vi "GenerateStimulusOutputs_Optogenetics.vi"(0 "Trial duration (min)":dbl, 1 "Rest duration(s)":dbl, 2 "trial offset (s)":dbl, 3 "Left Pad":dbl, 4 "Right Pad":dbl, 5 "Auditory":dbl, 6 "LED":dbl, 8 "LED Stim Duration (s)":dbl, 9 "LED Stim Parameters":cluster{"Fs":dbl, "Samples":dbl}, 10 "LED Frequency":dbl, 11 "Sol Stim Parameters":cluster{"Fs":dbl, "Samples":dbl}, 12 "LED duty cycle (%)":dbl, 14 "Sol Stim Duration (s)":dbl, 16 "Sol Frequency":dbl, 18 "Sol Duty Cycle (%)":dbl) -> (15 "Double LED Out":dbl[](array[numeric]), 20 "Solenoid Stim Waveforms":digitalwaveform(graph), 22 "Stimulus Digital Outputs":digitalwaveform[](array[waveform]), 24 "Left Pad Out":digitalwaveform(graph), 25 "Auditory Out":digitalwaveform(graph), 26 "Right Pad Out":digitalwaveform(graph), 27 "LED Out":digitalwaveform(graph))   [LabVIEW 2018]
uses:
  <vilib>/Waveform/DWDTOps.llb/DWDT Analog to Digital.vi
  <vilib>/Waveform/DWDTOps.llb/DWDT Digital to Analog.vi
  <vilib>/measure/NI_MABase.lvlib
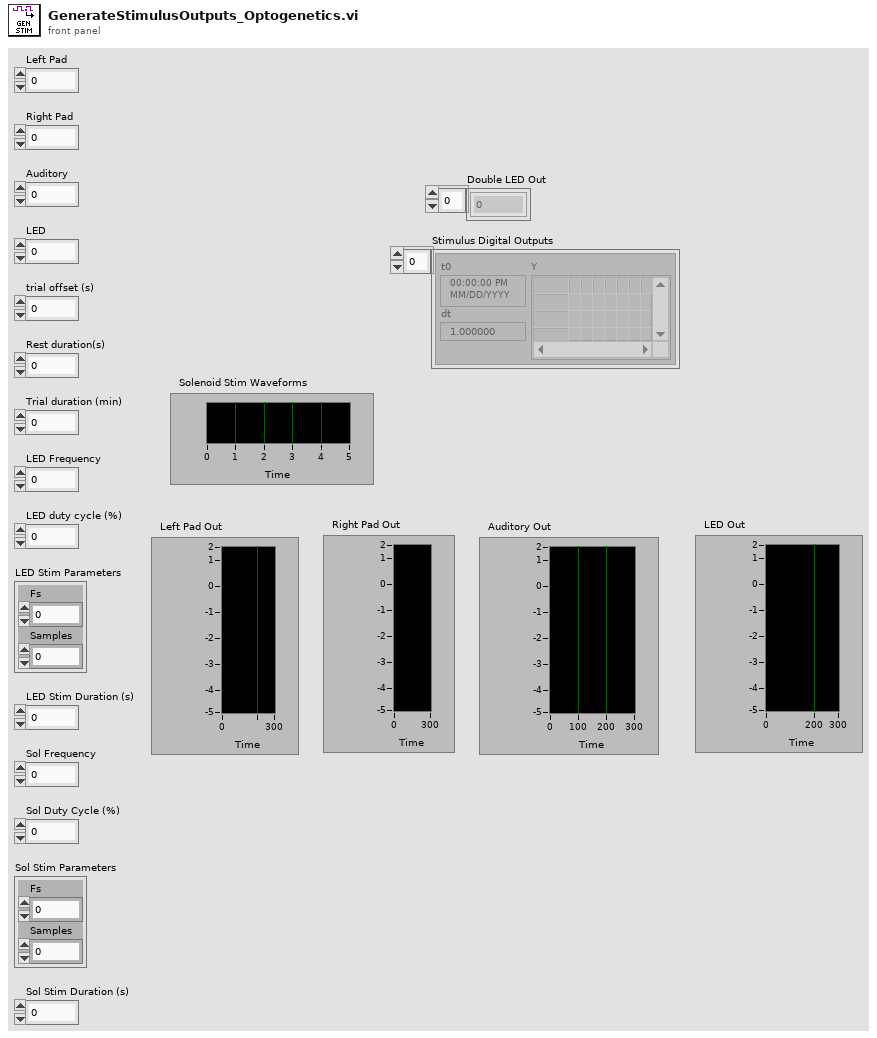
[diagram p1: front panel]
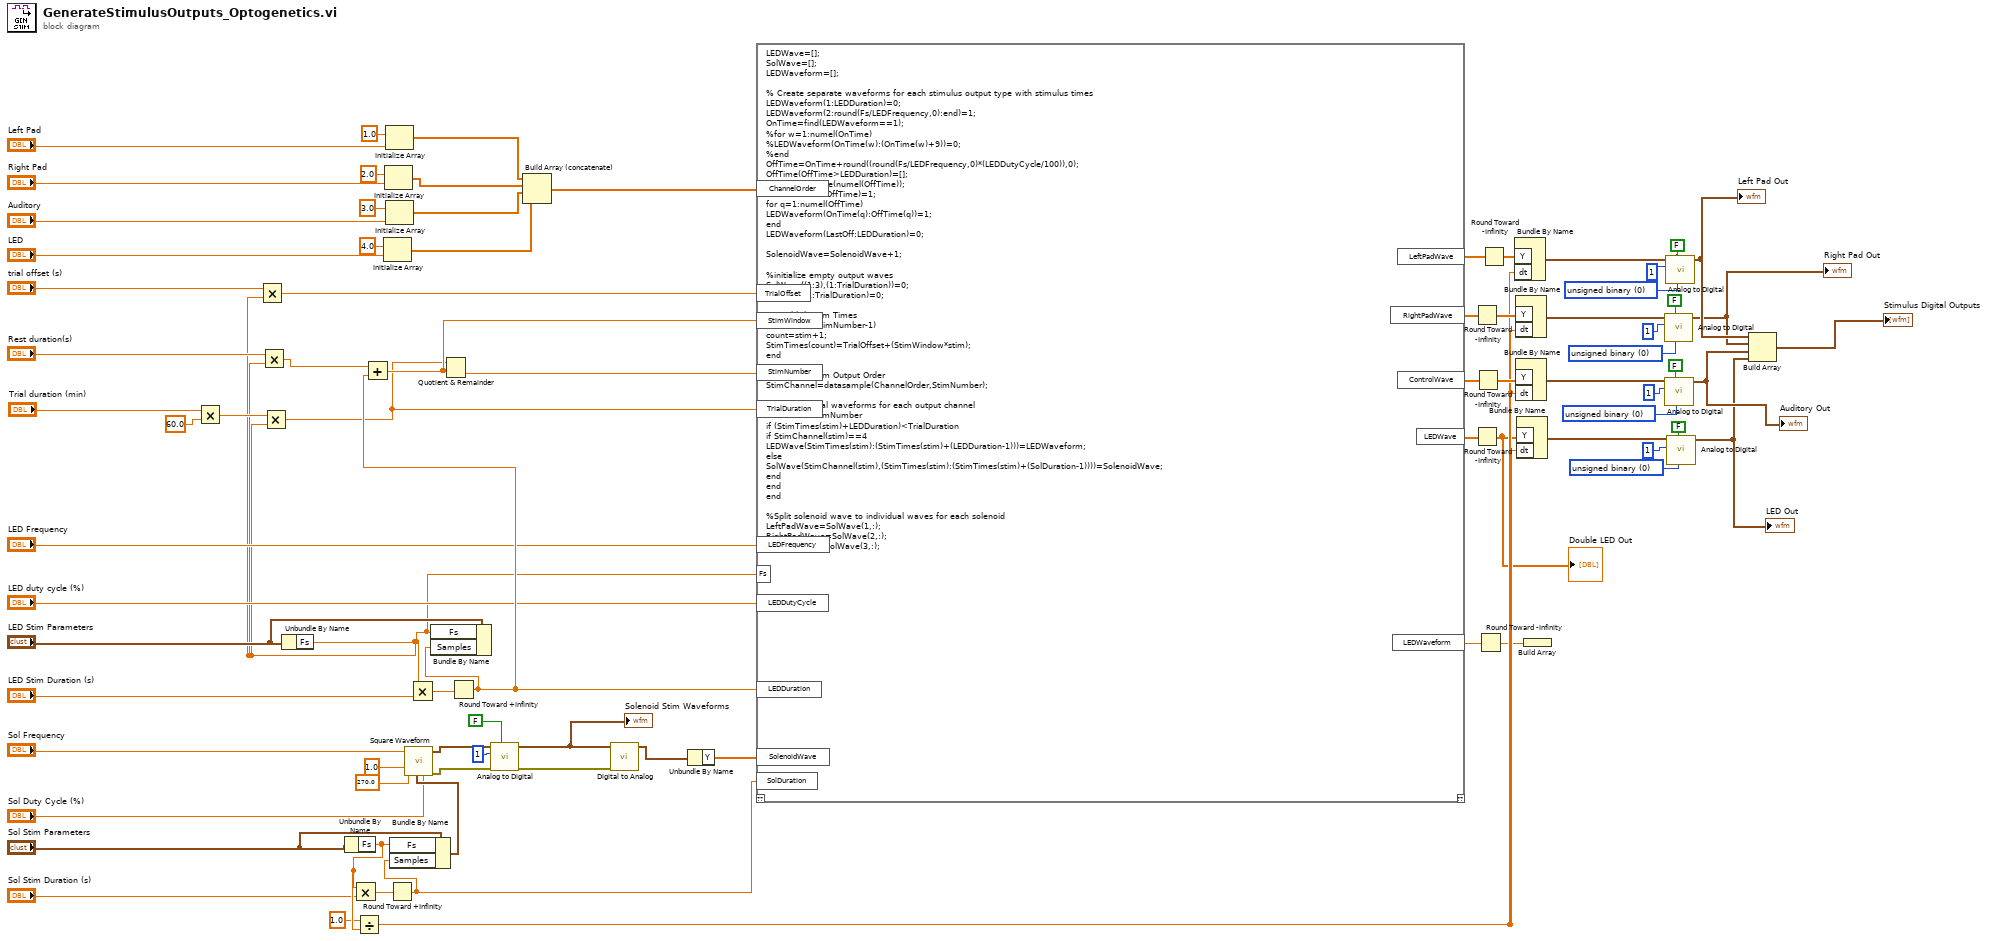
[diagram p0: block diagram]
diagram:
  w78 = u16 0 items=["unsigned binary", "offset binary", "2's complement"] ("data format (offset binary)")
  w77 = u16 0 items=["unsigned binary", "offset binary", "2's complement"] ("data format (offset binary)")
  w76 = u16 0 items=["unsigned binary", "offset binary", "2's complement"] ("data format (offset binary)")
  w75 = u16 0 items=["unsigned binary", "offset binary", "2's complement"] ("data format (offset binary)")
  n1 = Multiply(x="Trial duration (min)", y=60.0) -> (x*y=w16:dbl)
  n2 = Unbundle By Name("LED Stim Parameters") -> ("Fs"=w8:dbl)
  n3 = Multiply(x="trial offset (s)", y=w8) -> (x*y=w63:dbl)
  n4 = Multiply(x="Rest duration(s)", y=w8) -> (x*y=w20:dbl)
  n5 = Multiply(x=w16, y=w8) -> (x*y=w4:dbl)
  n6 = Unbundle By Name("Sol Stim Parameters") -> ("Fs"=w68:dbl)
  n7 = Multiply(x=w68, y="Sol Stim Duration (s)") -> (x*y=w50:dbl)
  n8 = Divide(x=1.0, y=w68) -> (x/y=w7:dbl)
  n9 = Initialize Array(4.0 ("element"), "LED") -> (w32:dbl[])
  n10 = Initialize Array(2.0 ("element"), "Right Pad") -> (w30:dbl[])
  n11 = Initialize Array(1.0 ("element"), "Left Pad") -> (w29:dbl[])
  n12 = Initialize Array(3.0 ("element"), "Auditory") -> (w31:dbl[])
  n13 = Round Toward +Infinity(x=w50) -> (ceil(x): smallest int >= x=w51:dbl)
  n14 = Bundle By Name(cluster="Sol Stim Parameters", "Fs"=w68, "Samples"=w51) -> (w38:cluster{"Fs":dbl, "Samples":dbl})
  n15 = call <vilib>:"Square Waveform.vi"("duty cycle (%)"="Sol Duty Cycle (%)", "sampling info"=w38, "phase"=270.0, "amplitude"=1.0, "frequency"="Sol Frequency") -> ("error out"=w41:errorcluster, "signal out"=w44:waveform(dbl))  [unwired: 5 in]
  n16 = Multiply(x=w8, y="LED Stim Duration (s)") -> (x*y=w49:dbl)
  n17 = Round Toward +Infinity(x=w49) -> (ceil(x): smallest int >= x=w80:dbl)
  n18 = Add(x=w20, y=w80) -> (x+y=w64:dbl)
  n19 = Bundle By Name(cluster="LED Stim Parameters", "Fs"=w8, "Samples"=w80) -> ()  [unwired: 1 out]
  n20 = Quotient & Remainder(x=w4, y=w64) -> (floor(x/y)=w61:dbl)  [unwired: 1 out]
  n21 = call-poly <vilib>:"Analog to Digital.vi"("compress digital (T)"=FALSE, "error in (no error)"=w41, "resolution (16 bit)"=1, "analog waveform"=w44) -> ("error out"=w42:errorcluster, "digital waveform"=w66:digitalwaveform)  [unwired: 4 in, 2 out]
  "Solenoid Stim Waveforms" <- w66
  n22 = Build Array (concatenate)(w29, w30, w31, w32) -> (w62:dbl[])
  n23 = call-poly <vilib>:"Digital to Analog.vi"("error in (no error)"=w42, "digital waveform"=w66) -> ("analog waveform"=w40:waveform(dbl))  [unwired: 6 in, 3 out]
  n24 = Unbundle By Name(w40) -> ("Y"=w60:dbl[])
  n25 = script code="LEDWave=[];\nSolWave=[];\nLEDWaveform=[];\n\n% Create separate waveforms for each stimulus output type with stimulus times\nLEDWaveform(1:LEDDuration)=0;\nLEDWaveform(2:round(Fs/LEDFrequency,0):end)=1;\nOnTime=find(LEDWaveform==1);\n%for w=1:numel(OnTime)\n%LEDWaveform(OnTime(w):(OnTime(w)+9))=0;\n%end\nOffTime=OnTime+round((round(Fs/LEDFrequency,0)*(LEDDutyCycle/100)),0);\nOffTime(OffTime>LEDDuration)=[];\nLastOff=OffTime(numel(OffTime));\nLEDWaveform(OffTime)=1;\nfor q=1:numel(OffTime)\nLEDWaveform(OnTime(q):OffTime(q))=1;\nend\nLEDWaveform(LastOff:LEDDuration)=0;\n\nSolenoidWave=SolenoidWave+1;\n\n%initialize empty output waves\nSolWave((1:3),(1:TrialDuration))=0;\nLEDWave(1:TrialDuration)=0;\n\n%Establish Stim Times\nfor stim=0:(StimNumber-1)\ncount=stim+1;\nStimTimes(count)=TrialOffset+(StimWindow*stim);\nend\n\n%Establish Stim Output Order\nStimChannel=datasample(ChannelOrder,StimNumber); \n\n% Compile trial waveforms for each output channel\nfor stim=1:StimNumber\nif (StimTimes(stim)+LEDDuration)<TrialDuration\nif StimChannel(stim)==4\nLEDWave(StimTimes(stim):(StimTimes(stim)+(LEDDuration-1)))=LEDWaveform;\nelse \nSolWave(StimChannel(stim),(StimTimes(stim):(StimTimes(stim)+(SolDuration-1))))=SolenoidWave;\nend\nend\nend\n\n%Split solenoid wave to individual waves for each solenoid\nLeftPadWave=SolWave(1,:);\nRightPadWave=SolWave(2,:);\nControlWave=SolWave(3,:);"("StimNumber"=w61, "ChannelOrder"=w62, "TrialDuration"=w4, "SolenoidWave"=w60, "LEDDuration"=w80, "SolDuration"=w51, "TrialOffset"=w63, "StimWindow"=w64, "LEDDutyCycle"="LED duty cycle (%)", "LEDFrequency"="LED Frequency", "Fs"=w8) -> ("LeftPadWave"=w81:dbl[], "RightPadWave"=w58:dbl[], "ControlWave"=w59:dbl[], "LEDWave"=w72:dbl[], "LEDWaveform"=w2:dbl)  [unwired: 1 in, 1 out]
  n26 = Round Toward -Infinity(1:w58) -> (0:w70:dbl[])
  n27 = Round Toward -Infinity(1:w72) -> (0:w3:dbl[])
  "Double LED Out" <- w3
  n28 = Round Toward -Infinity(1:w59) -> (0:w71:dbl[])
  n29 = Round Toward -Infinity(1:w2) -> (0:w1:dbl)
  n30 = Round Toward -Infinity(1:w81) -> (0:w69:dbl[])
  n31 = Bundle By Name("Y"=w69, "dt"=w7) -> (w6:waveform(dbl))  [unwired: 1 in]
  n32 = Bundle By Name("Y"=w70, "dt"=w7) -> (w79:waveform(dbl))  [unwired: 1 in]
  n33 = Bundle By Name("Y"=w71, "dt"=w7) -> (w74:waveform(dbl))  [unwired: 1 in]
  n34 = Bundle By Name("Y"=w3, "dt"=w7) -> (w73:waveform(dbl))  [unwired: 1 in]
  n35 = Build Array(w1) -> ()  [unwired: 1 out]
  n36 = call-poly <vilib>:"Analog to Digital.vi"("data format (offset binary)"=w76, "compress digital (T)"=FALSE, "resolution (16 bit)"=1, "analog waveform"=w79) -> ("digital waveform"=w12:digitalwaveform)  [unwired: 4 in, 3 out]
  "Right Pad Out" <- w12
  n37 = call-poly <vilib>:"Analog to Digital.vi"("data format (offset binary)"=w77, "compress digital (T)"=FALSE, "resolution (16 bit)"=1, "analog waveform"=w74) -> ("digital waveform"=w11:digitalwaveform)  [unwired: 4 in, 3 out]
  "Auditory Out" <- w11
  n38 = call-poly <vilib>:"Analog to Digital.vi"("data format (offset binary)"=w75, "compress digital (T)"=FALSE, "resolution (16 bit)"=1, "analog waveform"=w6) -> ("digital waveform"=w13:digitalwaveform)  [unwired: 4 in, 3 out]
  "Left Pad Out" <- w13
  n39 = call-poly <vilib>:"Analog to Digital.vi"("data format (offset binary)"=w78, "compress digital (T)"=FALSE, "resolution (16 bit)"=1, "analog waveform"=w73) -> ("digital waveform"=w5:digitalwaveform)  [unwired: 4 in, 3 out]
  "LED Out" <- w5
  n40 = Build Array(w13, w12, w11, w5) -> (→"Stimulus Digital Outputs":digitalwaveform[])
